vi "TDMS.SetMetadata.vi"(8 "error in (no error)":errorcluster, 9 "DUTs":bool[](array[boolean])=[FALSE, FALSE, FALSE, FALSE, FALSE, FALSE, FALSE, FALSE, FALSE], 10 "LVTransitionParameters":T2={"ODH"={"Level"=1.0, "Band"=0.5, "TimeTolerance"=0.095}, "OPH.Duty"={"Level"=65.0, "Band"=10.0, "TimeTolerance"=0.095}, "OPH.Freq"={"Level"=100.0, "Band"=10.0, "TimeTolerance"=0.095}}, 11 "TestMetaData":T1) -> (0 "error out":errorcluster)   [LabVIEW 2015, in "TestStand Utilities.lvlib"]
uses:
  TestStand Utilities.lvlib
  Shared/Public.LVAnalysis.ctl
  Shared/Public.ChLVAnalysis.ctl
  Shared/Constants.vi
  Shared/Shared.lvlib
panel:
  in  "DUTs.SN":string[](array[string])
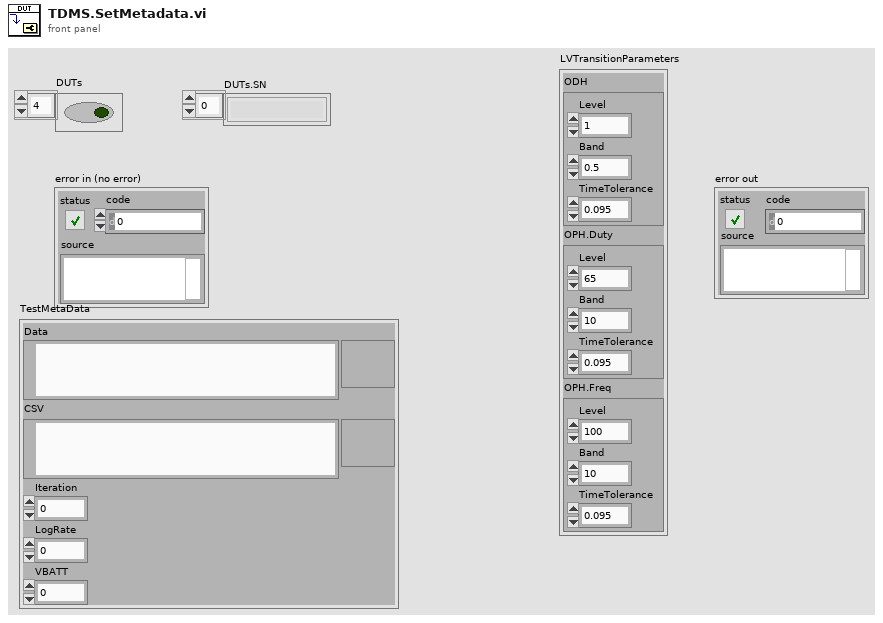
[diagram p1: front panel]
types:
  T1 = cluster{"Data":path, "CSV":path, "Iteration":i32, "LogRate":dbl, "VBATT":dbl}
  T2 = typedef "Shared.lvlib/Public.LVAnalysis.ctl" = cluster{"ODH":T3, "OPH.Duty":T3, "OPH.Freq":T3}
  T3 = typedef "Shared.lvlib/Public.ChLVAnalysis.ctl" = cluster{"Level":dbl, "Band":dbl, "TimeTolerance":dbl}
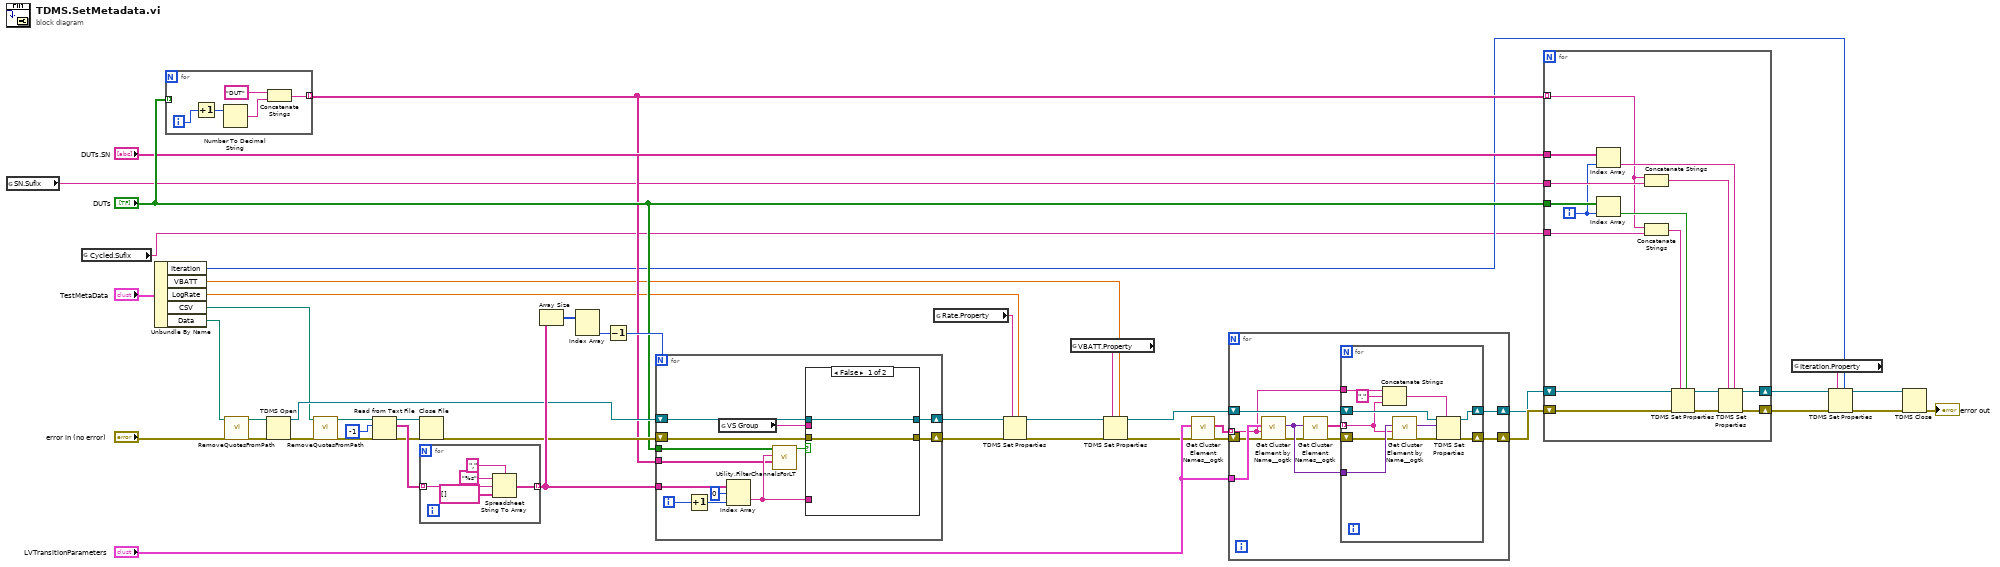
[diagram p0: block diagram]
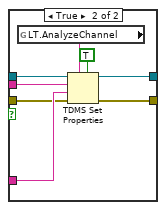
[diagram p2: hidden frame]
diagram:
  n1 = global read "Constants.vi" "SN.Sufix"() -> (w2:string)
  n2 = global read "Constants.vi" "Cycled.Sufix"() -> (w1:string)
  n3 = Unbundle By Name("TestMetaData") -> ("Iteration"=w16:i32, "VBATT"=w15:dbl, "LogRate"=w14:dbl, "CSV"=w13:path, "Data"=w11:path)
  n4 = for {
    tunnel: "DUTs" -> [_] mode=indexing
    tunnel: [w47] -> w18 mode=indexing
    i -> [w48]
    n5 = Increment(x=w48) -> (x+1=w50:i32)
    n6 = Number To Decimal String(number=w50) -> (decimal integer string=w49:string)  [unwired: 1 in]
    n7 = Concatenate Strings("DUT", w49) -> (w47:string)
  }
  n8 = call "RemoveQuotesFromPath.vi"("error in (no error)"="error in (no error)", "Data"=w11) -> ("error out"=w7:errorcluster, "Path"=w10:path)  [unwired: 8 in]
  n9 = TDMS Open(8:w7, 11:w10) -> (0:w9:errorcluster, 3:w29:refnum<k34>)  [unwired: 5 in]
  n10 = call "RemoveQuotesFromPath.vi"("error in (no error)"=w9, "Data"=w13) -> ("error out"=w8:errorcluster, "Path"=w12:path)  [unwired: 8 in]
  n11 = Read from Text File(file (use dialog)=w12, count=-1, error in=w8) -> (refnum out=w35:refnum<file>, text=w36:string[], error out=w34:errorcluster)  [unwired: 1 in, 1 out]
  n12 = Close File(refnum=w35, error in=w34) -> (error out=w30:errorcluster)  [unwired: 1 out]
  n13 = for {
    tunnel: w36 -> [w56] mode=indexing
    tunnel: [w52] -> w31 mode=indexing
    n14 = Spreadsheet String To Array(delimiter (Tab)=",", format string="%s", spreadsheet string=w56, array type (2D Dbl)=string[] []) -> (array=w52:string[])
  }
  n15 = Array Size(array=w31) -> (size(s)=w38:i32[])
  n16 = Index Array(array=w38) -> (element #2=w37:i32)  [unwired: 2 in, 1 out]
  n17 = Decrement(x=w37) -> (x-1=w32:i32)
  n18 = for {
    N: w32 -> [_]
    tunnel: w31 -> [w67]
    tunnel: "DUTs" -> [w60]
    shift-right: [w65] -> w27
    shift-left: w29 -> [w64]
    shift-right: [w63] -> w28
    shift-left: w30 -> [w62]
    tunnel: w18 -> [w57]
    i -> [w68]
    n19 = Increment(x=w68) -> (x+1=w69:i32)
    n20 = global read "Constants.vi" "VS Group"() -> (w61:string)
    n21 = Index Array(array=w67, index (row)=0 ("disabled index (row)"), index (col)=w69) -> (element=w58:string)
    n22 = call "Utility.FilterChannelsForLT.vi"(9:"DUTs"=w57, "Channel"=w58, 11:"DUTs"=w60) -> ("Use?"=w59:bool)  [unwired: 7 in, 1 out]
    n23 = case shown="False" w59 {
      tunnel: w58 -> [_ w79]
      tunnel: [w71 w77] -> w65
      tunnel: w64 -> [w71 w76]
      tunnel: [w70 w75] -> w63
      tunnel: w62 -> [w70 w74]
      tunnel: w61 -> [_ w73]
      frame False {
      }
      frame True {
        n24 = global read "Constants.vi" "LT.AnalyzeChannel"() -> (w72:string)
        n25 = TDMS Set Properties(5:TRUE, 7:w72, 8:w74, 9:w79, 10:w73, 11:w76) -> (0:w75:errorcluster, 3:w77:refnum<k34>)  [unwired: 2 out]
      }
    }
  }
  n26 = global read "Constants.vi" "Rate.Property"() -> (w5:string)
  n27 = TDMS Set Properties(5:w14, 7:w5, 8:w28, 11:w27) -> (0:w26:errorcluster, 3:w25:refnum<k34>)  [unwired: 2 in, 2 out]
  n28 = global read "Constants.vi" "VBATT.Property"() -> (w4:string)
  n29 = TDMS Set Properties(5:w15, 7:w4, 8:w26, 11:w25) -> (0:w40:errorcluster, 3:w39:refnum<k34>)  [unwired: 2 in, 2 out]
  n30 = call <userlib>:"Get Cluster Element Names__ogtk.vi"("error in (no error)"=w40, "Cluster"="LVTransitionParameters") -> ("error out"=w41:errorcluster, "Element Names"=w43:string[])  [unwired: 8 in]
  n31 = for {
    shift-right: [w89] -> w45
    shift-left: w41 -> [w85]
    shift-right: [w87] -> w44
    shift-left: w39 -> [w88]
    tunnel: w43 -> [w80] mode=indexing
    tunnel: "LVTransitionParameters" -> [w86]
    n32 = call <userlib>:"Get Cluster Element by Name__ogtk.vi"("error in (no error)"=w85, "Element Name"=w80, "Cluster"=w86) -> ("error out"=w82:errorcluster, "VElement"=w84:variant)  [unwired: 6 in, 1 out]
    n33 = call <userlib>:"Get Cluster Element Names__ogtk.vi"("error in (no error)"=w82, "Cluster"=w84) -> ("error out"=w81:errorcluster, "Element Names"=w83:string[])  [unwired: 8 in]
    n34 = for {
      tunnel: w84 -> [w97]
      shift-right: [w98] -> w87
      shift-left: w88 -> [w99]
      shift-right: [w100] -> w89
      shift-left: w81 -> [w95]
      tunnel: w83 -> [w91] mode=indexing
      tunnel: w80 -> [w92]
      n35 = Concatenate Strings(w92, "." ("string"), w91) -> (w90:string)
      n36 = call <userlib>:"Get Cluster Element by Name__ogtk.vi"("error in (no error)"=w95, "Element Name"=w91, "Cluster"=w97) -> ("error out"=w94:errorcluster, "VElement"=w96:variant)  [unwired: 6 in, 1 out]
      n37 = TDMS Set Properties(5:w96, 7:w90, 8:w94, 11:w99) -> (0:w100:errorcluster, 3:w98:refnum<k34>)  [unwired: 2 in, 2 out]
    }
  }
  n38 = for {
    tunnel: w1 -> [w116]
    shift-right: [w102] -> w23
    shift-left: w44 -> [w115]
    shift-right: [w103] -> w24
    shift-left: w45 -> [w114]
    tunnel: "DUTs" -> [w108]
    tunnel: w2 -> [w110]
    tunnel: "DUTs.SN" -> [w106]
    tunnel: w18 -> [w101] mode=indexing
    i -> [w104]
    n39 = Index Array(array=w106, index=w104) -> (element=w105:string)
    n40 = Index Array(array=w108, index=w104) -> (element=w107:bool)
    n41 = Concatenate Strings(w101, w110) -> (w109:string)
    n42 = Concatenate Strings(w101, w116) -> (w111:string)
    n43 = TDMS Set Properties(5:w107, 7:w111, 8:w114, 11:w115) -> (0:w113:errorcluster, 3:w112:refnum<k34>)  [unwired: 2 in, 2 out]
    n44 = TDMS Set Properties(5:w105, 7:w109, 8:w113, 11:w112) -> (0:w103:errorcluster, 3:w102:refnum<k34>)  [unwired: 2 in, 2 out]
  }
  n45 = global read "Constants.vi" "Iteration.Property"() -> (w3:string)
  n46 = TDMS Set Properties(5:w16, 7:w3, 8:w24, 11:w23) -> (0:w22:errorcluster, 3:w21:refnum<k34>)  [unwired: 2 in, 2 out]
  n47 = TDMS Close(8:w22, 11:w21) -> (0:→"error out":errorcluster)  [unwired: 1 out]
